vi "t2ns.vi"(1 "t/div":T1(ring)) -> (0 "ns/div":u32)   [LabVIEW 2011]
doc: "Converts ns/div to a plain time (ns) value\neg. 10 us/div = 10000ns"
panel:
  # "=>"
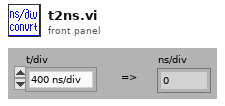
[diagram p1: front panel]
types:
  T1 = enum16{"400 ns/div", "1 us/div", "2 us/div", "4 us/div", "10 us/div", "20 us/div"}
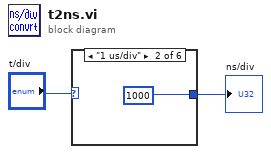
[diagram p0: block diagram]
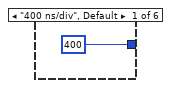
[diagram p2: hidden frame]
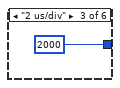
[diagram p3: hidden frame]
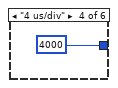
[diagram p4: hidden frame]
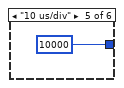
[diagram p5: hidden frame]
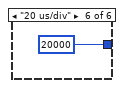
[diagram p6: hidden frame]
diagram:
  n1 = case shown="\"1 us/div\"" "t/div" {
    tunnel: [400 1000 2000 4000 10000 20000] -> w1
    frame "400 ns/div", Default {
    }
    frame "1 us/div" {
    }
    frame "2 us/div" {
    }
    frame "4 us/div" {
    }
    frame "10 us/div" {
    }
    frame "20 us/div" {
    }
  }
  "ns/div" <- w1
